vi "reposition.vi"() -> ()   [LabVIEW 2022 SP3]
panel:
  in  "20x":bool
  in  "Point of Interest - y":dbl
  in  "Point of Interest - x":dbl
  # "objective magnification"
  # "50x"
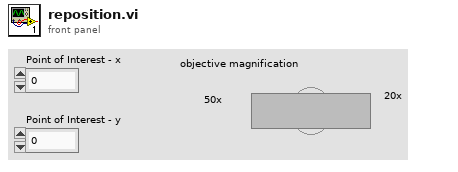
[diagram p1: front panel]
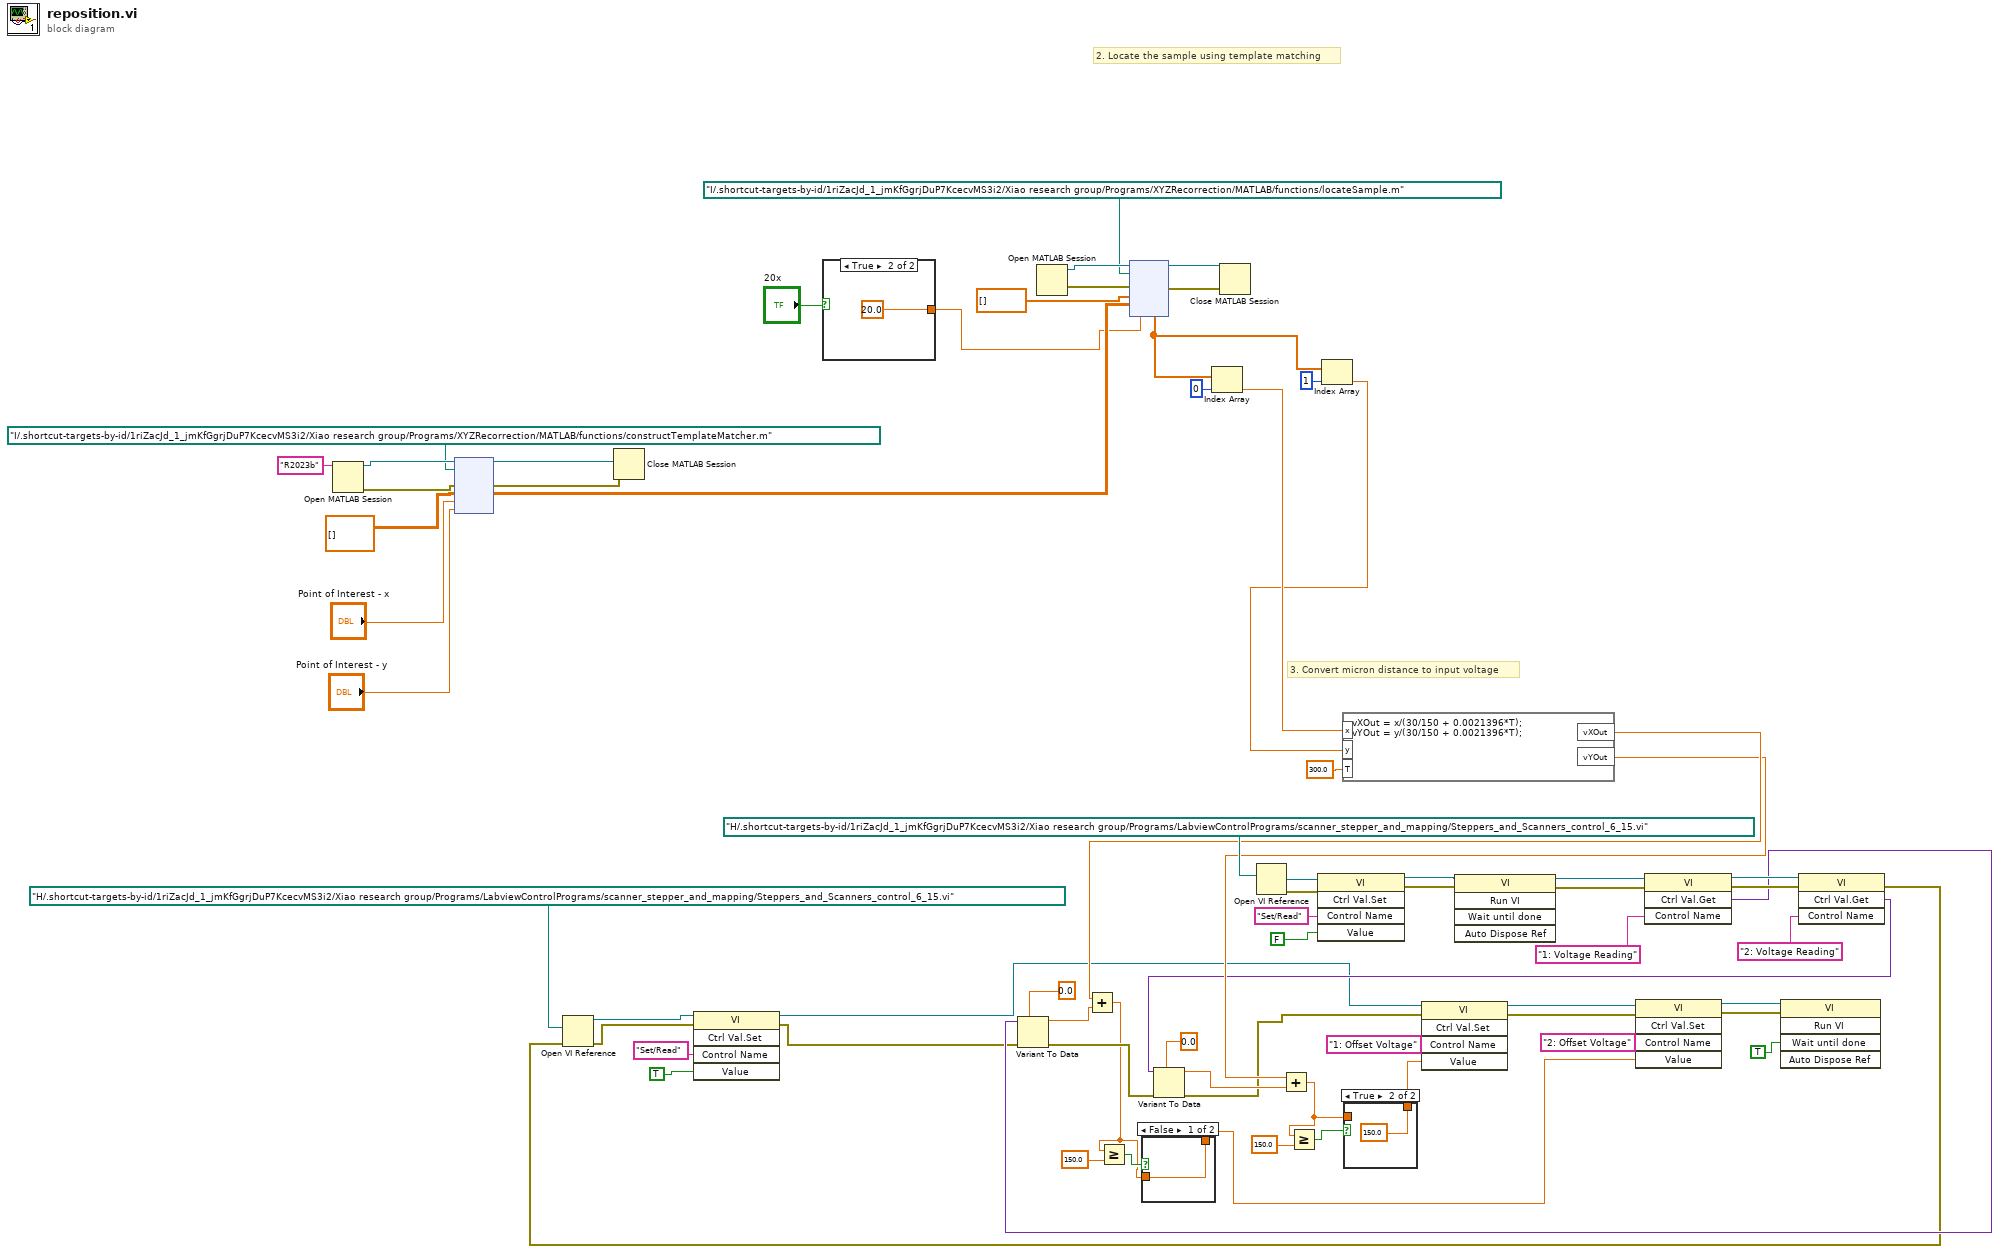
[diagram p0: block diagram]
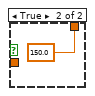
[diagram p2: hidden frame]
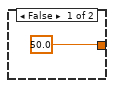
[diagram p4: hidden frame]
diagram:
  # "3. Convert micron distance to input voltage"
  # "2. Locate the sample using template matching"
  n1 = Open MATLAB Session(0:"R2023b" ("release name")) -> (8:w39:refnum<k37>, 11:w38:errorcluster)  [unwired: 1 in]
  n2 = node(w39, path "I:/.shortcut-targets-by-id/1riZacJd_1_jmKfGgrjDuP7KcecvMS3i2/Xiao research group/Programs/XYZRecorrection/MATLAB/functions/constructTemplateMatcher.m" ("source file path"), w38, dbl[][] [], "Point of Interest - x", "Point of Interest - y") -> (w33:refnum<k37>, w32:errorcluster, w25:dbl[][])  [unwired: 3 in, 2 out]
  n3 = Close MATLAB Session(0:w33, 3:w32) -> ()  [unwired: 1 out]
  n4 = case shown="True" "20x" {
    tunnel: [50.0 20.0] -> w9
    frame False {
    }
    frame True {
    }
  }
  n5 = Open MATLAB Session() -> (8:w30:refnum<k37>, 11:w27:errorcluster)  [unwired: 2 in]
  n6 = node(w30, path "I:/.shortcut-targets-by-id/1riZacJd_1_jmKfGgrjDuP7KcecvMS3i2/Xiao research group/Programs/XYZRecorrection/MATLAB/functions/locateSample.m" ("source file path"), w27, dbl[] [], w25, w9) -> (w29:refnum<k37>, w28:errorcluster, w22:dbl[])  [unwired: 3 in, 2 out]
  n7 = Index Array(array=w22, index=0 ("index (row)")) -> (element=w21:dbl)
  n8 = Close MATLAB Session(0:w29, 3:w28) -> ()  [unwired: 1 out]
  n9 = Open VI Reference(vi path=path "H:/.shortcut-targets-by-id/1riZacJd_1_jmKfGgrjDuP7KcecvMS3i2/Xiao research group/Programs/LabviewControlPrograms/scanner_stepper_and_mapping/Steppers_and_Scanners_control_6_15.vi") -> (vi reference=w62:refnum<vi>, error out=w61:errorcluster)  [unwired: 5 in]
  n10 = invoke class="VI" method="Ctrl Val.Set"(reference=w62, error in=w61, "Control Name"="Set/Read", "Value"=FALSE ("Wait Until Done")) -> (reference out=w60:refnum<vi>, error out=w59:errorcluster)  [unwired: 1 in, 3 out]
  n11 = Index Array(array=w22, index=1 ("index (row)")) -> (element=w20:dbl)
  n12 = formula code="vXOut = x/(30/150 + 0.0021396*T);\nvYOut = y/(30/150 + 0.0021396*T);"("x"=w21, "y"=w20, "T"=300.0 ("input variable")) -> ("vXOut"=w48:dbl, "vYOut"=w44:dbl)
  n13 = invoke class="VI" method="Run VI"(reference=w60, error in=w59) -> (reference out=w56:refnum<vi>, error out=w55:errorcluster)  [unwired: 3 in, 3 out]
  n14 = invoke class="VI" method="Ctrl Val.Get"(reference=w56, error in=w55, "Control Name"="1: Voltage Reading") -> (reference out=w53:refnum<vi>, error out=w52:errorcluster, "Get Control Value Variant"=w50:variant)  [unwired: 1 in, 1 out]
  n15 = invoke class="VI" method="Ctrl Val.Get"(reference=w53, error in=w52, "Control Name"="2: Voltage Reading") -> (error out=w17:errorcluster, "Get Control Value Variant"=w42:variant)  [unwired: 1 in, 2 out]
  n16 = Open VI Reference(vi path=path "H:/.shortcut-targets-by-id/1riZacJd_1_jmKfGgrjDuP7KcecvMS3i2/Xiao research group/Programs/LabviewControlPrograms/scanner_stepper_and_mapping/Steppers_and_Scanners_control_6_15.vi", error in (no error)=w17) -> (vi reference=w14:refnum<vi>, error out=w13:errorcluster)  [unwired: 4 in]
  n17 = invoke class="VI" method="Ctrl Val.Set"(reference=w14, error in=w13, "Control Name"="Set/Read", "Value"=TRUE ("Wait Until Done")) -> (reference out=w12:refnum<vi>, error out=w11:errorcluster)  [unwired: 1 in, 3 out]
  n18 = Variant To Data(error in=w11, type=0.0, Variant=w50) -> (data=w47:dbl, error out=w43:errorcluster)
  n19 = Add(x=w48, y=w47) -> (x+y=w1:dbl)
  n20 = Greater Or Equal?(x=w1, y=150.0) -> (x >= y?=w3:bool)
  n21 = case shown="False" w3 {
    tunnel: [w73 150.0 ("y")] -> w2
    tunnel: w1 -> [w73 _]
    frame False {
    }
    frame True {
    }
  }
  n22 = Variant To Data(error in=w43, type=0.0, Variant=w42) -> (data=w45:dbl, error out=w41:errorcluster)
  n23 = Add(x=w44, y=w45) -> (x+y=w5:dbl)
  n24 = Greater Or Equal?(x=w5, y=150.0) -> (x >= y?=w7:bool)
  n25 = case shown="True" w7 {
    tunnel: [w75 150.0 ("y")] -> w6
    tunnel: w5 -> [w75 _]
    frame False {
    }
    frame True {
    }
  }
  n26 = invoke class="VI" method="Ctrl Val.Set"(reference=w12, error in=w41, "Control Name"="1: Offset Voltage", "Value"=w6) -> (reference out=w67:refnum<vi>, error out=w68:errorcluster)  [unwired: 1 in, 3 out]
  n27 = invoke class="VI" method="Ctrl Val.Set"(reference=w67, error in=w68, "Control Name"="2: Offset Voltage", "Value"=w2) -> (reference out=w69:refnum<vi>, error out=w70:errorcluster)  [unwired: 1 in, 3 out]
  n28 = invoke class="VI" method="Run VI"(reference=w69, error in=w70, "Wait until done"=TRUE ("Wait Until Done")) -> ()  [unwired: 2 in, 5 out]
